vi "Read Model Number.vi"(8 "error in (no error)":errorcluster, 11 "UUT in":refnum<class "UUT.lvclass">) -> (0 "error out":errorcluster, 2 "Model Number":string, 3 "UUT out":refnum<class "UUT.lvclass">)   [LabVIEW 2021, in "Sequence Engine.lvlib" / "UUT.lvclass"]
uses:
  UUT.lvclass
  UUT.lvclass/UUT.ctl
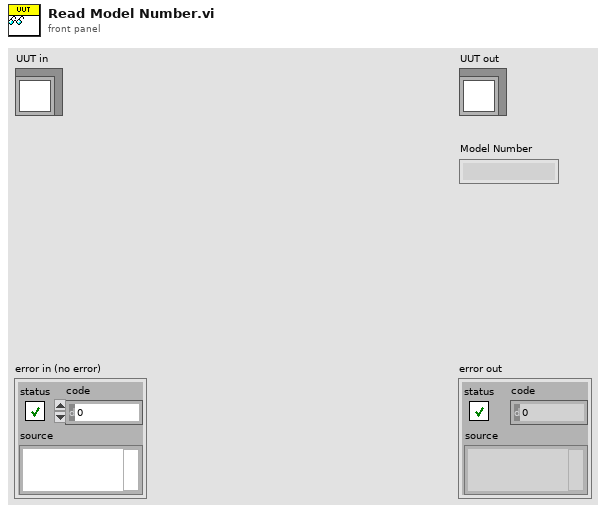
[diagram p1: front panel]
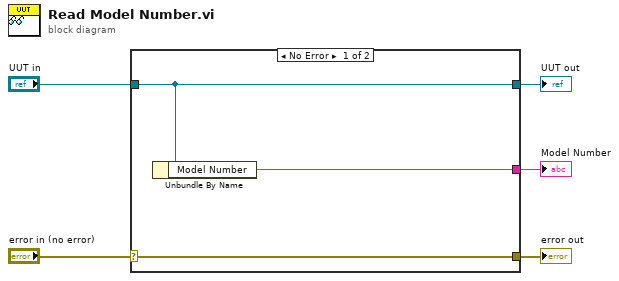
[diagram p0: block diagram]
diagram:
  n1 = case shown="No Error" "error in (no error)" {
    selector: "error in (no error)" -> [w8 w9]
    tunnel: [w8 w9] -> w4
    tunnel: [w7 w10] -> w2
    tunnel: "UUT in" -> [w7 w10]
    tunnel: [w6 _] -> w1
    frame No Error {
      n2 = Unbundle By Name(w7) -> ("Model Number"=w6:string)
    }
    frame Error {
    }
  }
  "error out" <- w4
  "UUT out" <- w2
  "Model Number" <- w1
